vi "MAIN_CALLED.vi"(8 "Error In":errorcluster, 11 "SESION VISA":refnum<visa-resource-name>="COM4") -> (0 "Error Out":errorcluster)   [LabVIEW 2019]
uses:
  TYPE'S DEF/INPUT_TRASPASO_ASICS.ctl
  LVPROJ_CONFIG_ESTACION/Type_defs/Coordenadas_estacion.ctl
  LVPROJ_CREAR BANDEJAS/Type_defs/Data_Bandeja.ctl
  TYPE'S DEF/OUTPUTS_TRASPASO_ASICS.ctl
  TYPE'S DEF/Estados_TRASPASO.ctl
  LVPROJ_MOVIMIENTO_CABEZAL/LABVIEW_MOVIMIENTO/MOVIMIENTO CABEZAL/Typedefs/Comandos.ctl
  LVPROJ_MOVIMIENTO_CABEZAL/LABVIEW_MOVIMIENTO/MOVIMIENTO CABEZAL/Typedefs/Estados_arduino.ctl
  LVPROJ_LEER_QR/LABVIEW/TYPE'S DEF/State_QR.ctl
  <vilib>/Utility/error.llb/Error Cluster From Error Code.vi
  <vilib>/ErrorRing/Error Ring.xnode
  SHARED VI'S/SHARED VI'S.lvlib
panel:
  in  "Tab DEPURACION":enum32{"Page 1", "Page 2"}(tab)
  out "PING OK":bool
  out "FINAL ASICS??":bool
  out "Asics pendientes":u32
  out "trama datos":string
  out "Movimiento realizado?":bool
  out "Datos de estación devueltos":string
  out "Datos de traspaso devueltos":string
  in  "Tab Control":T1(tab)
  in  "ENVIAR INPUTS TRASPASO":bool
  in  "EXIT":bool
  in  "COMENZAR TRASPASO":bool
  out "INDICADORES DE TEST":T2
  in  "TRASPASO ASICS INPUT":T3
  out "ESTADO FSM":T4
  out "Configuracion Estación":T5={"Coordenadas_estacion"={"Coord.Bandeja entrada"={"Coord. X0 entrada"=0, "Coord. Y0 entrada "=0, "Altura Z entrada"=0}, "Coord.Bandeja OK"={"Coord. X0 OK"=0, "Coord. Y0 OK"=0, "Altura Z OK"=0}, "Coord.Bandeja entrada FAIL"={"Coord. X0 FAIL"=0, "Coord. Y0 FAIL"=0, "Altura Z FAIL"=0}, "Coord. Socket"={"Coord. X socket"=0, "Coord. Y socket"=0, "Altura Z socket"=0}}, "Nombre Bandeja"="", "Datos bandeja"={"Nº de columnas "=0, "Nº de filas "=0, "largo"=0, "ancho"=0, "nombre"="nombre", "Paso X (en mm)"=0.0, "Paso Y (en mm)"=0.0, "DISTANCIA SUELO A CHIP  "=0.0, "Nº de celdas totales"=0, "Distancia chips bandejas contiguas"=0.0}}
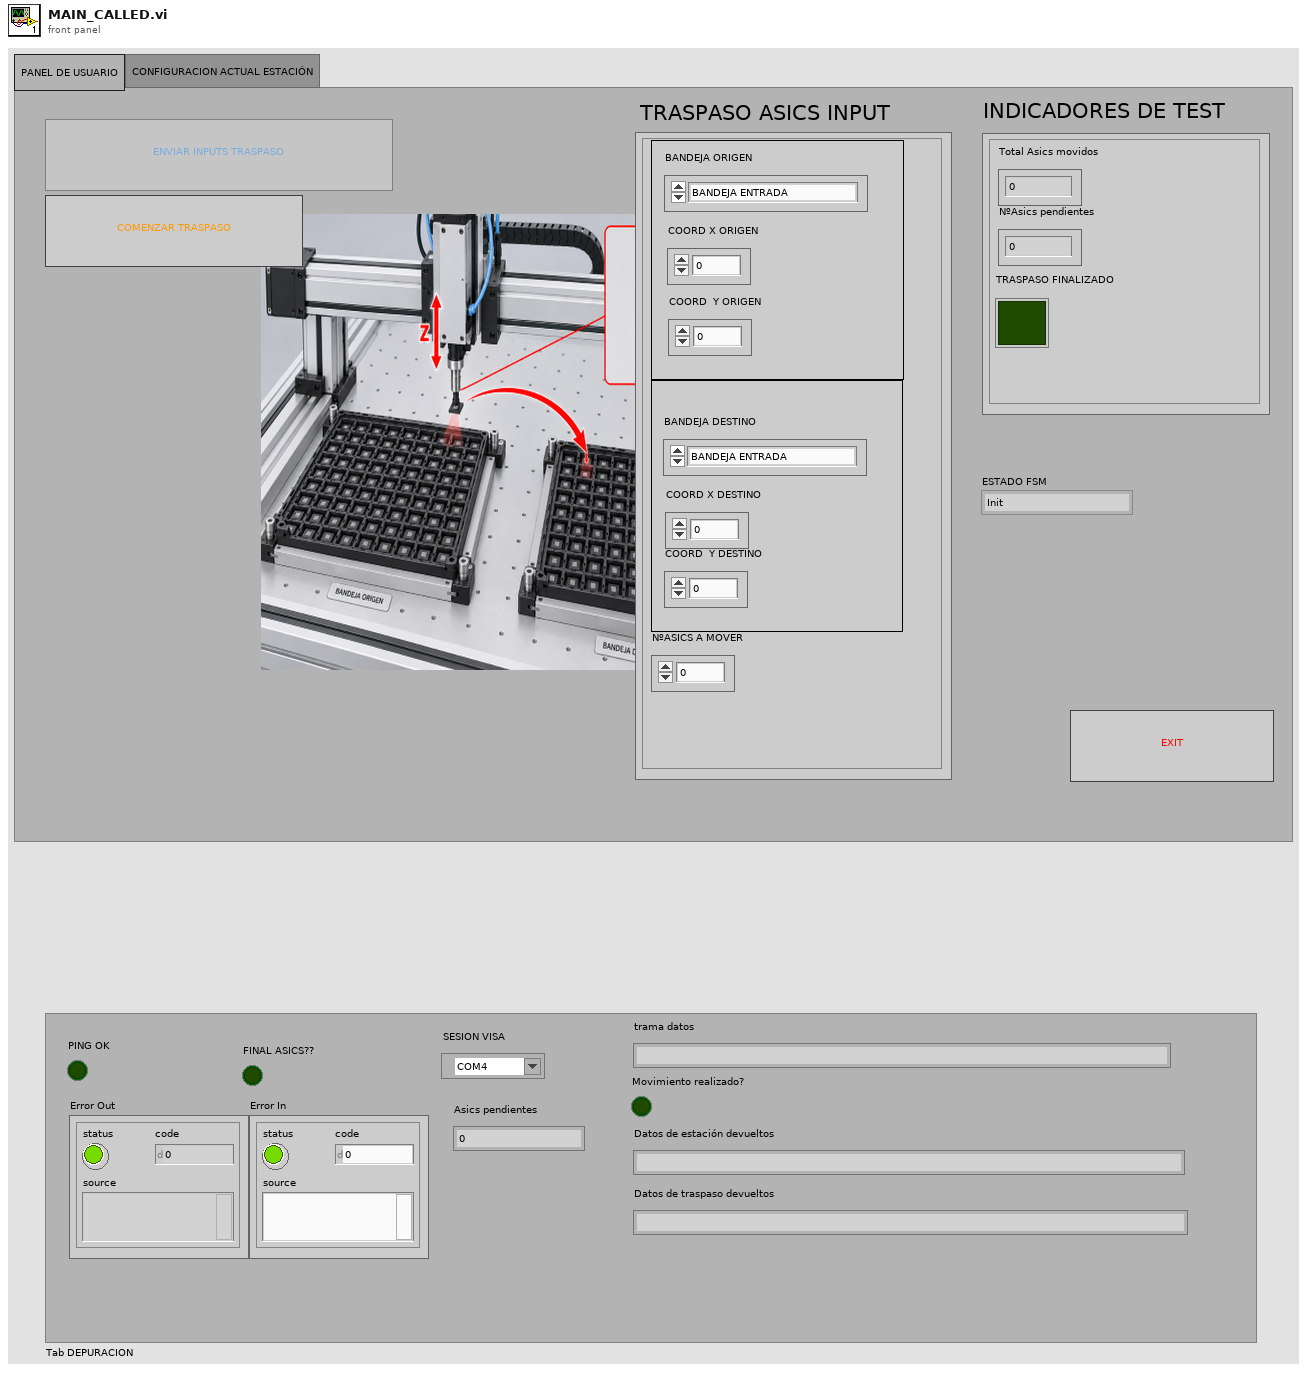
[diagram p1: front panel]
types:
  T1 = enum32{"PANEL DE USUARIO", "CONFIGURACION ACTUAL ESTACIÓN"}
  T2 = typedef "OUTPUTS_TRASPASO_ASICS.ctl" = cluster{"TRASPASO FINALIZADO":bool, "Total Asics movidos":u32, "NºAsics pendientes":u32}
  T3 = typedef "INPUT_TRASPASO_ASICS.ctl" = cluster{"COORD X ORIGEN":u32, "COORD  Y ORIGEN":u32, "NºASICS A MOVER":u32, "BANDEJA ORIGEN":enum16{"BANDEJA ENTRADA", "BANDEJA OK", "BANDEJA NOK"}, "BANDEJA DESTINO":enum16{"BANDEJA ENTRADA", "BANDEJA OK", "BANDEJA NOK"}, "COORD X DESTINO ":u32, "COORD  Y DESTINO ":u32, "CONTEO TRASLADOS":u32}
  T4 = typedef "Estados_TRASPASO.ctl" = enum16{"Init", "Wait for Event", "Init refs", "Init com", "Config estacion", "Introducir valores traspaso", "Home", "Ping_Arduino", "Esperar fin movimiento", "Enviar_config_test", "Actualizar valores", "Final traspaso?", "Terminar", "Exit", "Error?"}
  T5 = typedef "Configuracion_estación.ctl" = cluster{"Coordenadas_estacion":T6, "Nombre Bandeja":string, "Datos bandeja":T7}
  T6 = typedef "Coordenadas_estacion.ctl" = cluster{"Coord.Bandeja entrada":cluster{"Coord. X0 entrada":u32, "Coord. Y0 entrada ":u32, "Altura Z entrada":u32}, "Coord.Bandeja OK":cluster{"Coord. X0 OK":u32, "Coord. Y0 OK":u32, "Altura Z OK":u32}, "Coord.Bandeja entrada FAIL":cluster{"Coord. X0 FAIL":u32, "Coord. Y0 FAIL":u32, "Altura Z FAIL":u32}, "Coord. Socket":cluster{"Coord. X socket":u32, "Coord. Y socket":u32, "Altura Z socket":u32}}
  T7 = typedef "Data_Bandeja.ctl" = cluster{"Nº de columnas ":u32, "Nº de filas ":u32, "largo":u32, "ancho":u32, "nombre":string, "Paso X (en mm)":dbl, "Paso Y (en mm)":dbl, "DISTANCIA SUELO A CHIP  ":dbl, "Nº de celdas totales":u16, "Distancia chips bandejas contiguas":dbl}
  T8 = enum8{"Enabled", "Disabled", "Disabled and Grayed Out"}
  T9 = typedef "Estados_arduino.ctl" = enum16{"2", "3", "4", "5", "6", "7", "9", "8"}
  T10 = typedef "Comandos.ctl" = enum16{"H", "FH", "FM", "FI", "FX", "FY", "FZ", "I", "OK"}
  T11 = enum16{"BANDEJA ENTRADA", "BANDEJA OK", "BANDEJA NOK"}
  T12 = typedef "State_QR.ctl" = enum16{"Init", "Wait for Event", "Init refs", "Init com", "Config estacion", "Home", "Ping_Arduino", "Coge Asic", "Enviar_config_test", "Dejar Asic", "Leer QR", "Actualizar valores", "Enviar OK Arduino", "Final de lecturas?", "Terminar", "Exit", "Error?"}
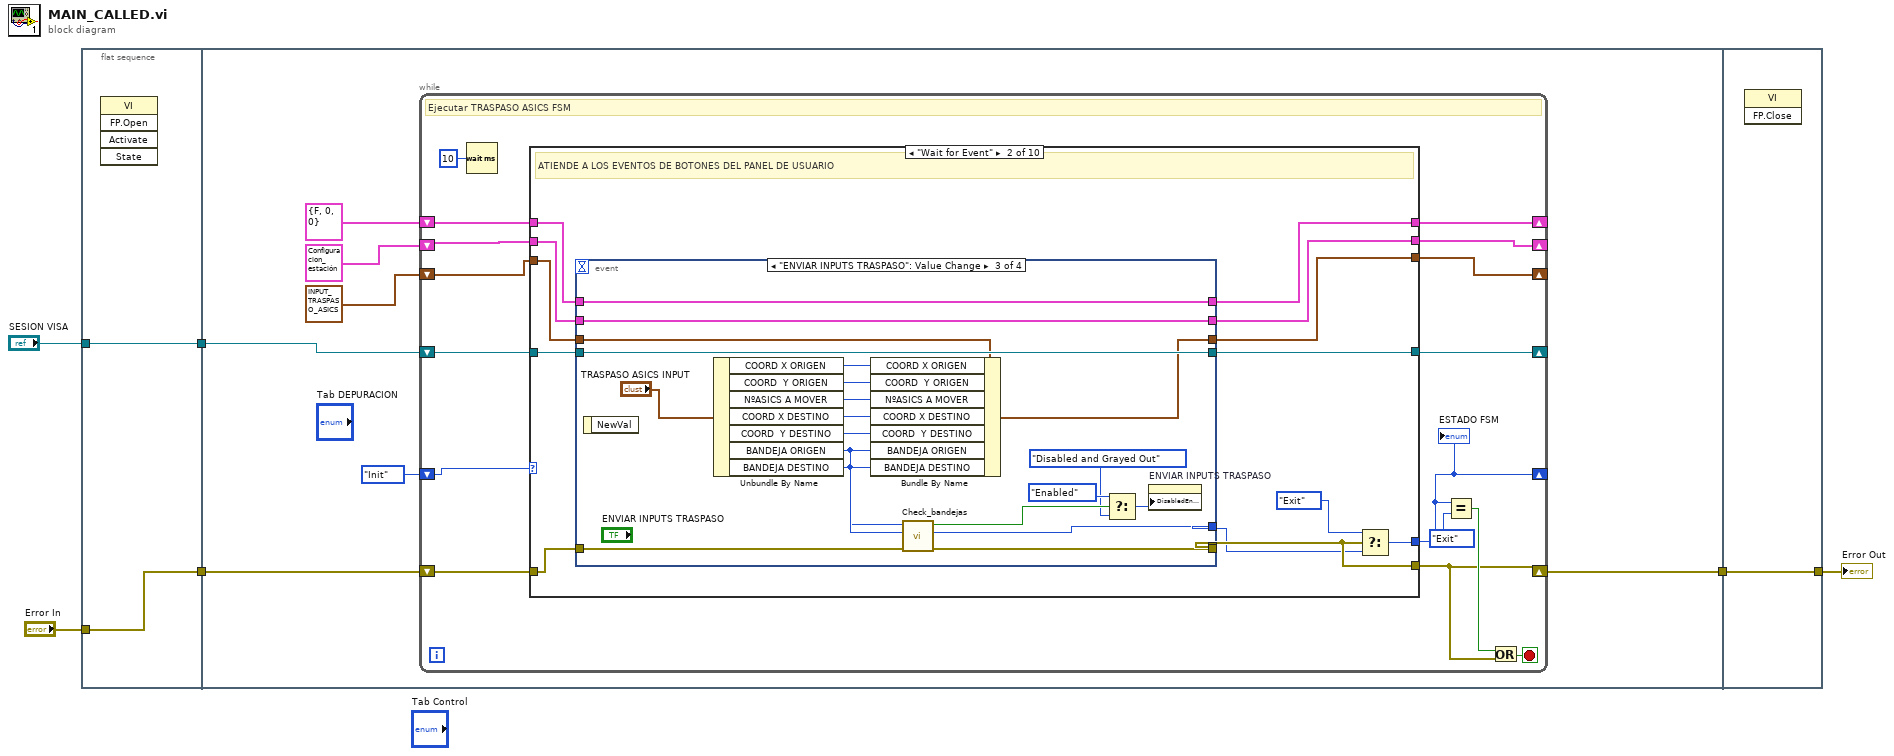
[diagram p0: block diagram]
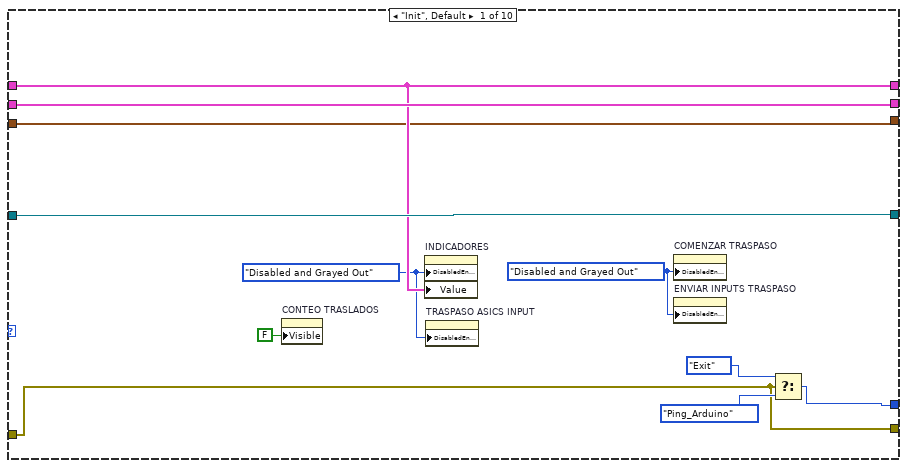
[diagram p2: hidden frame]
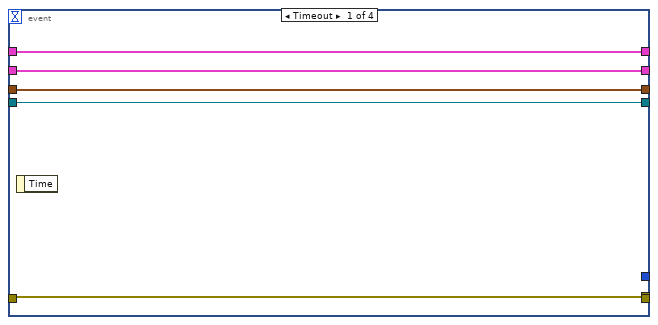
[diagram p3: hidden frame]
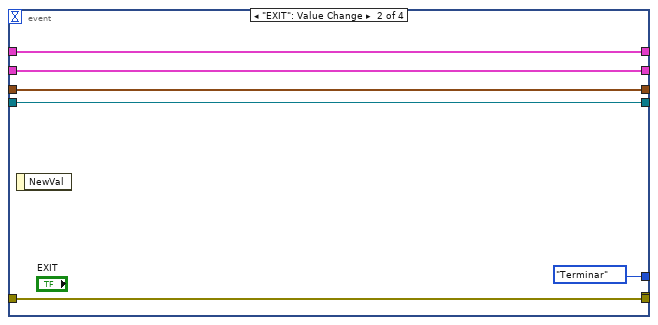
[diagram p4: hidden frame]
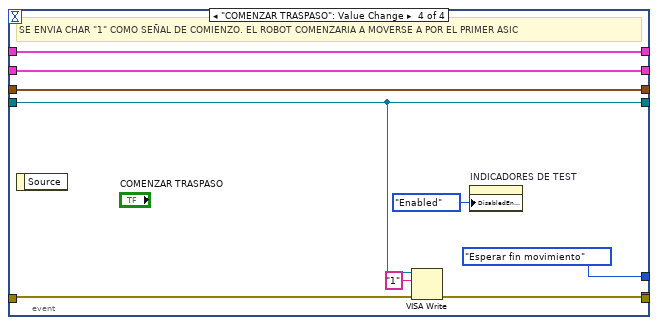
[diagram p5: hidden frame]
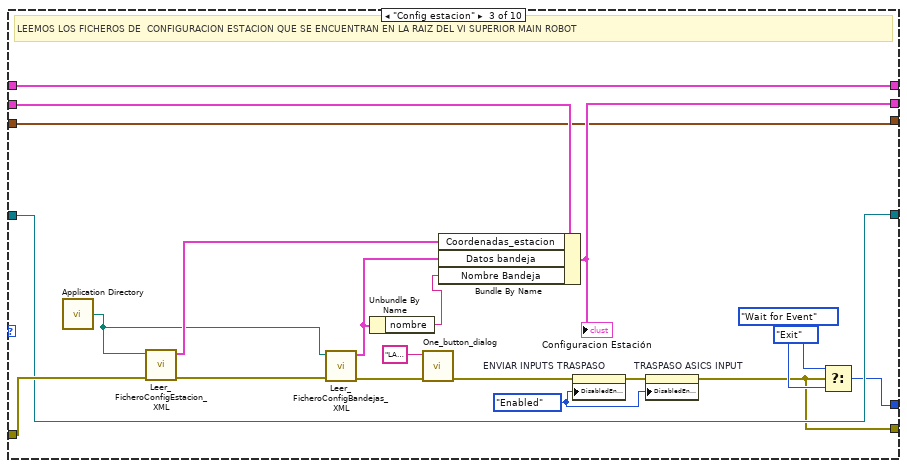
[diagram p6: hidden frame]
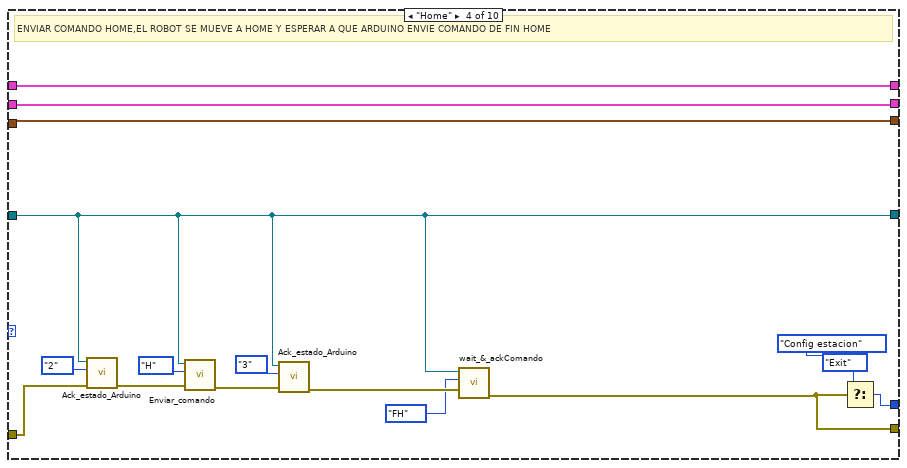
[diagram p7: hidden frame]
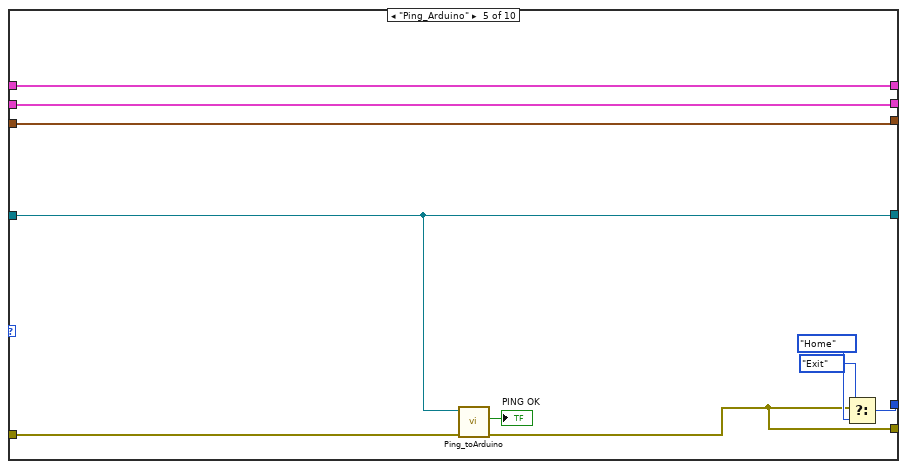
[diagram p8: hidden frame]
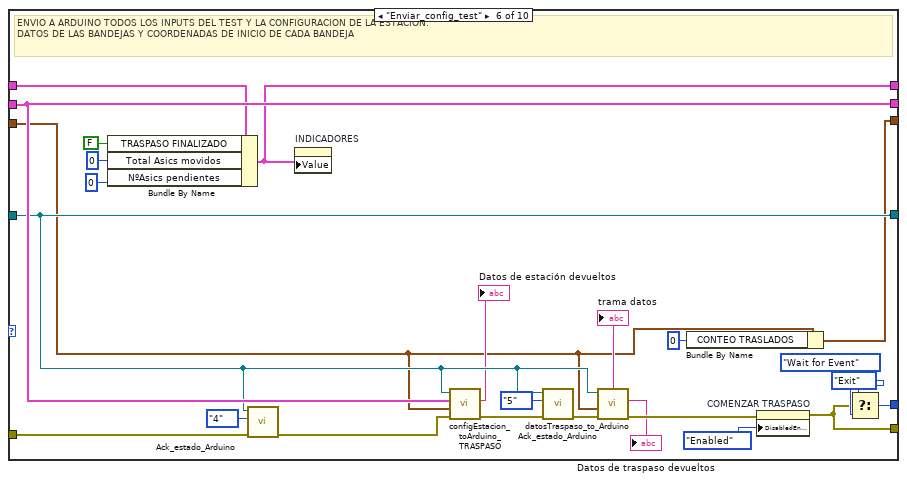
[diagram p9: hidden frame]
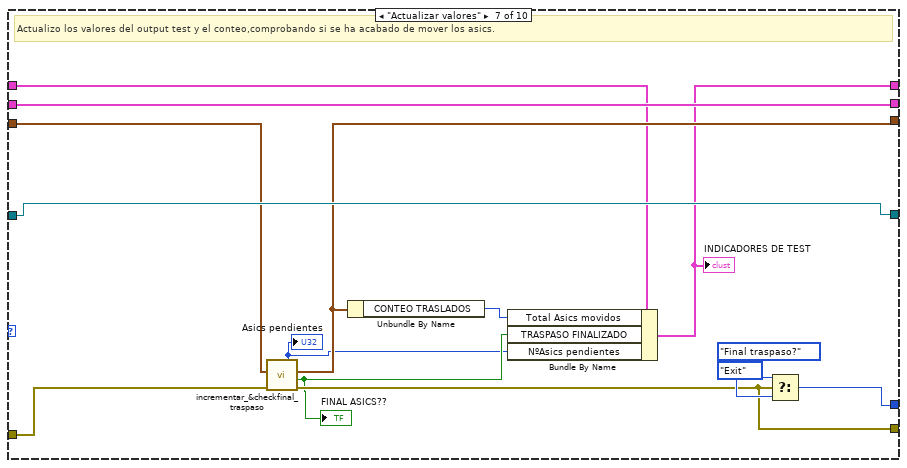
[diagram p10: hidden frame]
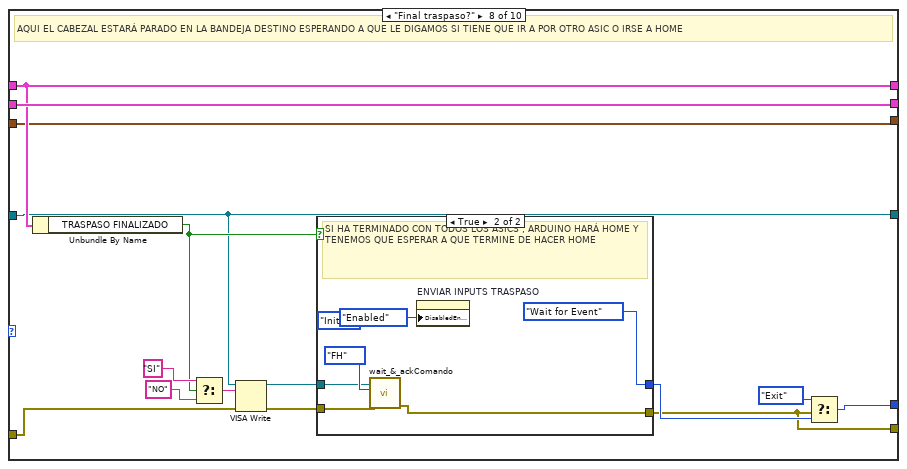
[diagram p11: hidden frame]
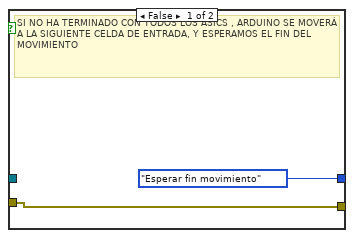
[diagram p12: hidden frame]
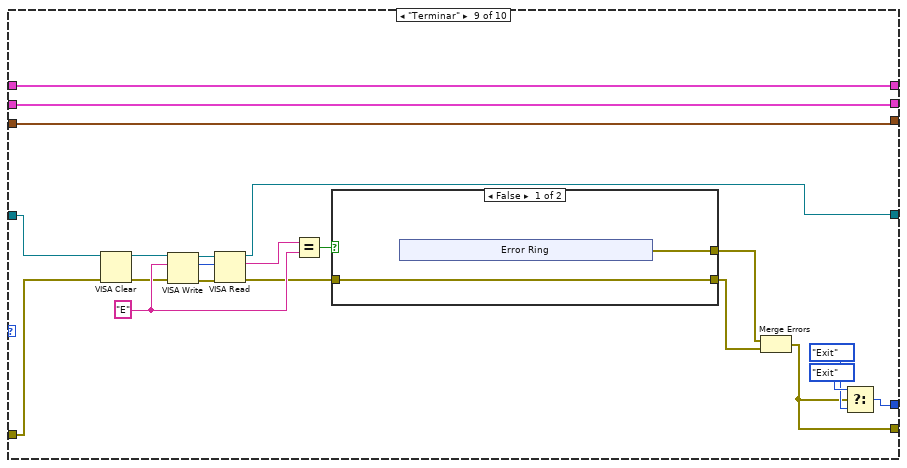
[diagram p13: hidden frame]
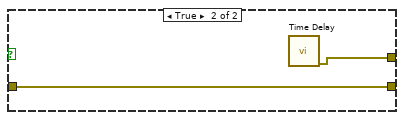
[diagram p14: hidden frame]
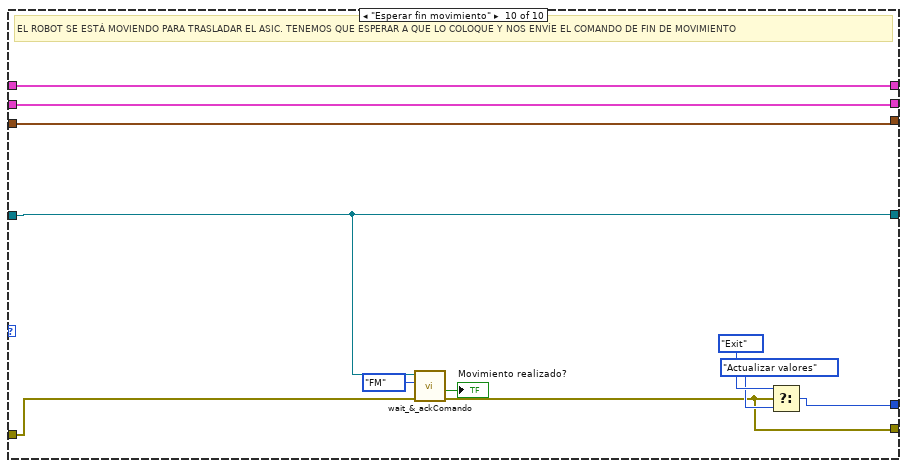
[diagram p15: hidden frame]
diagram:
  n1 = flat-sequence {
    tunnel: "Error In" -> [w8]
    tunnel: [w8] -> w6
    tunnel: "SESION VISA" -> [w7]
    tunnel: [w7] -> w4
    tunnel: w6 -> [w13]
    tunnel: w4 -> [w10]
    tunnel: [w9] -> w2
    tunnel: w2 -> [w245]
    tunnel: [w245] -> w1
    frame #0 {
      n2 = invoke class="VI" method="FP.Open"() -> ()  [unwired: 5 in, 5 out]
    }
    frame #1 {
      n3 = while {
        shift-right: [w26] -> w9
        shift-left: w13 -> [w30]
        shift-right: [w19] -> _
        shift-left: T3 {"COORD X ORIGEN"=0, "COORD  Y ORIGEN"=0, "NºASICS A MOVER"=1, "BANDEJA ORIGEN"=enum."BANDEJA ENTRADA", "BANDEJA DESTINO"=enum."BANDEJA ENTRADA", "COORD X DESTINO "=0, "COORD  Y DESTINO "=0, "CONTEO TRASLADOS"=0} ("TEST ASICS INPUT") -> [w29]
        shift-right: [w21] -> _
        shift-left: T5 {"Coordenadas_estacion"={"Coord.Bandeja entrada"={"Coord. X0 entrada"=0, "Coord. Y0 entrada "=0, "Altura Z entrada"=0}, "Coord.Bandeja OK"={"Coord. X0 OK"=0, "Coord. Y0 OK"=0, "Altura Z OK"=0}, "Coord.Bandeja entrada FAIL"={"Coord. X0 FAIL"=0, "Coord. Y0 FAIL"=0, "Altura Z FAIL"=0}, "Coord. Socket"={"Coord. X socket"=0, "Coord. Y socket"=0, "Altura Z socket"=0}}, "Nombre Bandeja"="", "Datos bandeja"={"Nº de columnas "=0, "Nº de filas "=0, "largo"=0, "ancho"=0, "nombre"="nombre", "Paso X (en mm)"=0.0, "Paso Y (en mm)"=0.0, "DISTANCIA SUELO A CHIP  "=0.0, "Nº de celdas totales"=0, "Distancia chips bandejas contiguas"=0.0}} ("Configuracion Estación") -> [w25]
        shift-right: [w23] -> _
        shift-left: w10 -> [w24]
        shift-right: [w20] -> _
        shift-left: T2 {"TRASPASO FINALIZADO"=FALSE, "Total Asics movidos"=0, "NºAsics pendientes"=0} -> [w22]
        shift-right: [w17] -> _
        shift-left: Estados_TRASPASO."Init" ("States_main") -> [w18]
        stop <- w28 stop-if-true
        # "Ejecutar TRASPASO ASICS FSM"
        n4 = Wait (ms)(milliseconds to wait=u32 10) -> ()  [unwired: 1 out]
        n5 = case shown="\"Wait for Event\"" w18 {
          tunnel: w30 -> [w38 w49 w115 w122 w135 w164 w175 w187 w207 w241]
          tunnel: w29 -> [w33 w51 w105 w129 w139 w144 w173 w181 w222 w240]
          tunnel: [w38 w48 w98 w117 w134 w150 w174 w182 w210 w237] -> w26
          tunnel: w25 -> [w40 w53 w108 w130 w140 w163 w178 w193 w223 w239]
          tunnel: w24 -> [w39 w46 w109 w119 w133 w157 w177 w186 w209 w236]
          tunnel: [w39 w45 w109 w119 w133 w157 w177 w186 w211 w236] -> w23
          tunnel: w22 -> [w36 w55 w106 w131 w141 w155 w169 w192 w224 w238]
          tunnel: [w40 w52 w107 w130 w140 w163 w178 w193 w223 w239] -> w21
          tunnel: [w36 w54 w106 w131 w141 w146 w167 w192 w224 w238] -> w20
          tunnel: [w33 w50 w105 w129 w139 w142 w171 w181 w222 w240] -> w19
          tunnel: [w37 w43 w102 w116 w136 w161 w176 w194 w219 w242] -> w17
          frame "Init", Default {
            w35 = T8."Disabled and Grayed Out" ("Disabled")
            w34 = T8."Disabled and Grayed Out" ("Disabled")
            n6 = property on="CONTEO TRASLADOS" class="DigNum (strict)"("Visible"=FALSE) -> ()  [unwired: 2 in, 2 out]
            n7 = property on="INDICADORES" class="Clust (strict)"("DisabledEnum"=w34, "Value"=w36) -> ()  [unwired: 2 in, 2 out]
            n8 = property on="TRASPASO ASICS INPUT" class="Clust (strict)"("DisabledEnum"=w34) -> ()  [unwired: 2 in, 2 out]
            n9 = property on="COMENZAR TRASPASO" class="Bool"("DisabledEnum"=w35) -> ()  [unwired: 2 in, 2 out]
            n10 = property on="ENVIAR INPUTS TRASPASO" class="Bool"("DisabledEnum"=w35) -> ()  [unwired: 2 in, 2 out]
            n11 = Select(t=Estados_TRASPASO."Exit" ("States_main"), s=w38, f=Estados_TRASPASO."Ping_Arduino" ("States_main")) -> (s? t:f=w37:T4)
          }
          frame "Wait for Event" {
            # "ATIENDE A LOS EVENTOS DE BOTONES DEL PANEL DE USUARIO"
            n12 = event shown="[2] \"ENVIAR INPUTS TRASPASO\": Value Change" {
              selector: _ -> [_ _ _ _]
              dyn-events: _ -> [_ _ _ _]
              timeout: _ -> [_ _ _ _]
              tunnel: w55 -> [w60 w66 w86 w95]
              tunnel: [w60 w66 w86 w95] -> w54
              tunnel: w53 -> [w59 w65 w85 w94]
              tunnel: [w59 w65 w85 w94] -> w52
              tunnel: w51 -> [w58 w64 w77 w93]
              tunnel: [w58 w64 w76 w93] -> w50
              tunnel: w49 -> [w57 w61 w73 w91]
              tunnel: [w57 _ w67 w90] -> w48
              tunnel: w46 -> [w56 w62 w84 w92]
              tunnel: [w56 w62 w84 w92] -> w45
              tunnel: [_ Estados_TRASPASO."Terminar" ("States_main") w72 Estados_TRASPASO."Esperar fin movimiento" ("States_main")] -> w44
              tunnel: [_ w61 _ _] -> _
              event Timeout {
                n13 = event-data() -> ()  [unwired: 1 in, 1 out]
              }
              event "EXIT": Value Change {
                n14 = event-data() -> ()  [unwired: 1 in, 1 out]
              }
              event "ENVIAR INPUTS TRASPASO": Value Change {
                n15 = event-data() -> ()  [unwired: 1 in, 1 out]
                n16 = Unbundle By Name("TRASPASO ASICS INPUT") -> ("COORD X ORIGEN"=w82:u32, "COORD  Y ORIGEN"=w81:u32, "NºASICS A MOVER"=w80:u32, "COORD X DESTINO"=w79:u32, "COORD  Y DESTINO"=w78:u32, "BANDEJA ORIGEN"=w75:T11, "BANDEJA DESTINO"=w74:T11)
                n17 = Bundle By Name(cluster=w77, "COORD X ORIGEN"=w82, "COORD  Y ORIGEN"=w81, "NºASICS A MOVER"=w80, "COORD X DESTINO"=w79, "COORD  Y DESTINO"=w78, "BANDEJA ORIGEN"=w75, "BANDEJA DESTINO"=w74) -> (w76:T3)
                n18 = call "Check_bandejas.vi"("error in (no error)"=w73, "BANDEJA ORIGEN"=w75, "BANDEJA DESTINO"=w74) -> ("error out"=w67:errorcluster, "States_main"=w72:T4, "Datos incorrectos"=w71:bool)  [unwired: 6 in]
                n19 = Select(t=T8."Enabled" ("Disabled"), s=w71, f=T8."Disabled and Grayed Out") -> (s? t:f=w68:T8)
                n20 = property on="ENVIAR INPUTS TRASPASO" class="Bool"("DisabledEnum"=w68) -> ()  [unwired: 2 in, 2 out]
              }
              event "COMENZAR TRASPASO": Value Change {
                # "SE ENVIA CHAR \"1\" COMO SEÑAL DE COMIENZO. EL ROBOT COMENZARIA A MOVERSE A POR EL PRIMER ASIC"
                n21 = event-data() -> ()  [unwired: 1 in, 1 out]
                n22 = VISA Write(VISA resource name=w92, write buffer="1", error in (no error)=w91) -> (error out=w90:errorcluster)  [unwired: 2 out]
                n23 = property on="INDICADORES DE TEST" class="Clust (strict)"("DisabledEnum"=T8."Enabled" ("Disabled")) -> ()  [unwired: 2 in, 2 out]
              }
            }
            n24 = Select(t=Estados_TRASPASO."Exit" ("States_main"), s=w48, f=w44) -> (s? t:f=w43:T4)
          }
          frame "Config estacion" {
            w97 = T8."Enabled" ("Disabled")
            # "LEEMOS LOS FICHEROS DE  CONFIGURACION ESTACION QUE SE ENCUENTRAN EN LA RAIZ DEL VI SUPERIOR MAIN ROBOT"
            n25 = call <vilib>:"Application Directory.vi"() -> ("Application Directory"=w96:path)
            n26 = call "Leer_FicheroConfigEstacion_XML.vi"("error in (no error)"=w115, "XML File Path"=w96) -> ("error out"=w114:errorcluster, "Coordenadas_estacion"=w113:T6)  [unwired: 8 in]
            n27 = call "Leer_FicheroConfigBandejas_XML.vi"("error in (no error)"=w114, "XML File Path"=w96) -> ("error out"=w110:errorcluster, "Datos bandeja"=w112:T7)  [unwired: 8 in]
            n28 = Unbundle By Name(w112) -> ("nombre"=w111:string)
            n29 = call "One_button_dialog.vi"("error in (no error)"=w110, "message"="LA CONFIGURACION DE LA ESTACIÓN SE HA LEÍDO CORRECTAMENTE") -> ("error out"=w100:errorcluster)  [unwired: 9 in]
            n30 = Bundle By Name(cluster=w108, "Coordenadas_estacion"=w113, "Datos bandeja"=w112, "Nombre Bandeja"=w111) -> (w107:T5)
            "Configuracion Estación" <- w107
            n31 = property on="ENVIAR INPUTS TRASPASO" class="Bool"(error in=w100, "DisabledEnum"=w97) -> (error out=w99:errorcluster)  [unwired: 1 in, 1 out]
            n32 = property on="TRASPASO ASICS INPUT" class="Clust (strict)"(error in=w99, "DisabledEnum"=w97) -> (error out=w98:errorcluster)  [unwired: 1 in, 1 out]
            n33 = Select(t=Estados_TRASPASO."Exit" ("States_main"), s=w98, f=Estados_TRASPASO."Wait for Event" ("States_main")) -> (s? t:f=w102:T4)
          }
          frame "Home" {
            # "ENVIAR COMANDO HOME,EL ROBOT SE MUEVE A HOME Y ESPERAR A QUE ARDUINO ENVIE COMANDO DE FIN HOME"
            n34 = call "Ack_estado_Arduino.vi"("error in (no error)"=w122, "Enum"=Estados_arduino."2", "VISA resource name"=w119) -> ("error out"=w128:errorcluster)  [unwired: 6 in, 2 out]
            n35 = call "Enviar_comando.vi"("error in (no error)"=w128, "Enum"=Comandos."H", "VISA resource name"=w119) -> ("error out"=w123:errorcluster)  [unwired: 6 in, 2 out]
            n36 = call "Ack_estado_Arduino.vi"("error in (no error)"=w123, "Enum"=Estados_arduino."3", "VISA resource name"=w119) -> ("error out"=w124:errorcluster)  [unwired: 6 in, 2 out]
            n37 = call "wait_&_ackComando.vi"("error in (no error)"=w124, 10:Comandos."FH", "VISA Refnum in"=w119) -> ("error out"=w117:errorcluster)  [unwired: 7 in, 1 out]
            n38 = Select(t=Estados_TRASPASO."Exit" ("States_main"), s=w117, f=Estados_TRASPASO."Config estacion" ("States_main")) -> (s? t:f=w116:T4)
          }
          frame "Ping_Arduino" {
            n39 = call "Ping_toArduino.vi"("error in (no error)"=w135, "VISA Refnum in"=w133) -> ("error out"=w134:errorcluster, "PING OK"=→"PING OK":bool)  [unwired: 7 in, 1 out]
            n40 = Select(t=Estados_TRASPASO."Exit" ("States_main"), s=w134, f=Estados_TRASPASO."Home" ("States_main")) -> (s? t:f=w136:T4)
          }
          frame "Enviar_config_test" {
            # "ENVIO A ARDUINO TODOS LOS INPUTS DEL TEST Y LA CONFIGURACION DE LA ESTACIÓN:\nDATOS DE LAS BANDEJAS Y COORDENADAS DE INICIO DE CADA BANDEJA"
            n41 = Bundle By Name(cluster=w155, "TRASPASO FINALIZADO"=FALSE, "Total Asics movidos"=u32 0, "NºAsics pendientes"=u32 0) -> (w146:T2)
            n42 = call "Ack_estado_Arduino.vi"("error in (no error)"=w164, "Enum"=Estados_arduino."4", "VISA resource name"=w157) -> ("error out"=w160:errorcluster)  [unwired: 6 in, 2 out]
            n43 = property on="INDICADORES" class="Clust (strict)"("Value"=w146) -> ()  [unwired: 2 in, 2 out]
            n44 = call "configEstacion_toArduino_TRASPASO.vi"("error in (no error)"=w160, "TRASPASO ASICS INPUT"=w144, "Configuracion Estación"=w163, "VISA resource name"=w157) -> ("error IO"=w162:errorcluster, "Datos de estación devueltos"=→"Datos de estación devueltos":string)  [unwired: 5 in, 1 out]
            n45 = call "Ack_estado_Arduino.vi"("error in (no error)"=w162, "Enum"=Estados_arduino."5", "VISA resource name"=w157) -> ("error out"=w159:errorcluster)  [unwired: 6 in, 2 out]
            n46 = call "datosTraspaso_to_Arduino.vi"("error in (no error)"=w159, "TRASPASO ASICS INPUT"=w144, "VISA resource name"=w157) -> ("error IO"=w151:errorcluster, "trama datos devuelta"=→"Datos de traspaso devueltos":string, "trama datos enviada"=→"trama datos":string)  [unwired: 6 in]
            n47 = Bundle By Name(cluster=w144, "CONTEO TRASLADOS"=u32 0) -> (w142:T3)
            n48 = property on="COMENZAR TRASPASO" class="Bool"(error in=w151, "DisabledEnum"=T8."Enabled" ("Disabled")) -> (error out=w150:errorcluster)  [unwired: 1 in, 1 out]
            n49 = Select(t=Estados_TRASPASO."Exit" ("States_main"), s=w150, f=Estados_TRASPASO."Wait for Event" ("States_main")) -> (s? t:f=w161:T4)
          }
          frame "Actualizar valores" {
            # "Actualizo los valores del output test y el conteo,comprobando si se ha acabado de mover los asics."
            n50 = call "incrementar_&checkfinal_traspaso.vi"("error in (no error)"=w175, "TRASPASO ASICS INPUT"=w173) -> ("error out"=w174:errorcluster, "FINAL ASICS??"=w170:bool, "output cluster"=w171:T3, "Asics pendientes"=w168:u32)  [unwired: 6 in]
            "FINAL ASICS??" <- w170
            "Asics pendientes" <- w168
            n51 = Unbundle By Name(w171) -> ("CONTEO TRASLADOS"=w172:u32)
            n52 = Bundle By Name(cluster=w169, "Total Asics movidos"=w172, "TRASPASO FINALIZADO"=w170, "NºAsics pendientes"=w168) -> (w167:T2)
            "INDICADORES DE TEST" <- w167
            n53 = Select(t=Estados_TRASPASO."Exit" ("States_main"), s=w174, f=Estados_TRASPASO."Final traspaso?" ("States_main")) -> (s? t:f=w176:T4)
          }
          frame "Final traspaso?" {
            (unwired) State_QR."Init" ("States_main")
            # "AQUI EL CABEZAL ESTARÁ PARADO EN LA BANDEJA DESTINO ESPERANDO A QUE LE DIGAMOS SI TIENE QUE IR A POR OTRO ASIC O IRSE A HOME"
            n54 = Unbundle By Name(w192) -> ("TRASPASO FINALIZADO"=w188:bool)
            n55 = Select(t="SI", s=w188, f="NO") -> (s? t:f=w189:string)
            n56 = VISA Write(VISA resource name=w186, write buffer=w189, error in (no error)=w187) -> (VISA resource name out=w183:refnum<visa-resource-name>, error out=w185:errorcluster)  [unwired: 1 out]
            n57 = case shown="True" w188 {
              tunnel: w185 -> [w196 w202]
              tunnel: [Estados_TRASPASO."Esperar fin movimiento" ("States_main") Estados_TRASPASO."Wait for Event" ("States_main")] -> w184
              tunnel: [w196 w200] -> w182
              tunnel: w183 -> [_ w199]
              frame False {
                # "SI NO HA TERMINADO CON TODOS LOS ASICS , ARDUINO SE MOVERÁ A LA SIGUIENTE CELDA DE ENTRADA, Y ESPERAMOS EL FIN DEL MOVIMIENTO"
              }
              frame True {
                # "SI HA TERMINADO CON TODOS LOS ASICS , ARDUINO HARÁ HOME Y TENEMOS QUE ESPERAR A QUE TERMINE DE HACER HOME"
                n58 = call "wait_&_ackComando.vi"("error in (no error)"=w202, 10:Comandos."FH", "VISA Refnum in"=w199) -> ("error out"=w200:errorcluster)  [unwired: 7 in, 1 out]
                n59 = property on="ENVIAR INPUTS TRASPASO" class="Bool"("DisabledEnum"=T8."Enabled" ("Disabled")) -> ()  [unwired: 2 in, 2 out]
              }
            }
            n60 = Select(t=Estados_TRASPASO."Exit" ("States_main"), s=w182, f=w184) -> (s? t:f=w194:T4)
          }
          frame "Terminar" {
            w216 = "E" ("write buffer")
            n61 = VISA Clear(VISA resource name=w209, error in (no error)=w207) -> (VISA resource name out=w208:refnum<visa-resource-name>, error out=w206:errorcluster)
            n62 = VISA Write(VISA resource name=w208, write buffer=w216, error in (no error)=w206) -> (VISA resource name out=w212:refnum<visa-resource-name>, return count=w218:u32, error out=w213:errorcluster)
            n63 = VISA Read(VISA resource name=w212, byte count=w218, error in (no error)=w213) -> (VISA resource name out=w211:refnum<visa-resource-name>, read buffer=w217:string, error out=w205:errorcluster)  [unwired: 1 out]
            n64 = Equal?(x=w217, y=w216) -> (x = y?=w215:bool)
            n65 = case shown="False" w215 {
              tunnel: [w226 w233] -> w214
              tunnel: w205 -> [w225 w232]
              tunnel: [w225 w232] -> w204
              frame False {
                n66 = xnode "Error Ring"() -> ("error out"=w226:errorcluster)
              }
              frame True {
                n67 = call "Time Delay"() -> ("error out"=w233:errorcluster)  [unwired: 11 in]
              }
            }
            n68 = Merge Errors(w214, w204) -> (w210:errorcluster)
            n69 = Select(t=Estados_TRASPASO."Exit" ("y"), s=w210, f=Estados_TRASPASO."Exit" ("y")) -> (s? t:f=w219:T4)
          }
          frame "Esperar fin movimiento" {
            # "EL ROBOT SE ESTÁ MOVIENDO PARA TRASLADAR EL ASIC. TENEMOS QUE ESPERAR A QUE LO COLOQUE Y NOS ENVÍE EL COMANDO DE FIN DE MOVIMIENTO"
            n70 = call "wait_&_ackComando.vi"("error in (no error)"=w241, 10:Comandos."FM", "VISA Refnum in"=w236) -> ("error out"=w237:errorcluster, "Movimiento realizado?"=→"Movimiento realizado?":bool)  [unwired: 7 in]
            n71 = Select(t=Estados_TRASPASO."Exit" ("States_main"), s=w237, f=Estados_TRASPASO."Actualizar valores" ("States_main")) -> (s? t:f=w242:T4)
          }
        }
        "ESTADO FSM" <- w17
        n72 = Equal?(x=w17, y=Estados_TRASPASO."Exit") -> (x = y?=w31:bool)
        n73 = Or(x=w31, y=w26) -> (x .or. y?=w28:bool)
      }
    }
    frame #2 {
      n74 = invoke class="VI" method="FP.Close"() -> ()  [unwired: 3 in, 3 out]
    }
  }
  "Error Out" <- w1
